vi "ReadDataFromDatabase.vi"(9 "长度":i32=1, 10 "index":i32, 11 "recordset data":variant[][](array[variant])) -> (2 "一行记录":string[](array[string]), 3 "所有记录":string[][](array[string]))   [LabVIEW 2014]
uses:
  <vilib>/addons/database/_DB Variant To Data/Database Variant To Data.xnode
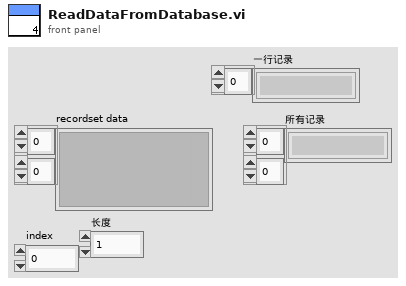
[diagram p1: front panel]
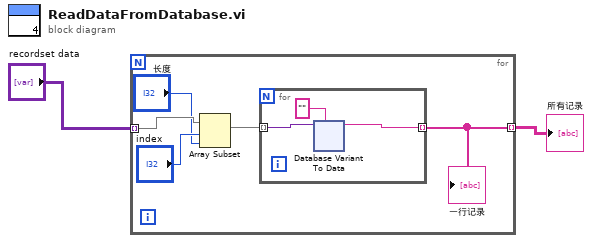
[diagram p0: block diagram]
diagram:
  n1 = for {
    tunnel: "recordset data" -> [w6] mode=indexing
    tunnel: [w5] -> w2 mode=indexing
    n2 = Array Subset(array=w6, index="index", length="长度") -> (w7:variant[])
    n3 = for {
      tunnel: w7 -> [w10] mode=indexing
      tunnel: [w8] -> w5 mode=indexing
      n4 = xnode "Database Variant To Data"("database variant"=w10, "type"="") -> ("data"=w8:string)  [unwired: 1 in, 1 out]
    }
    "一行记录" <- w5
  }
  "所有记录" <- w2
